vi "Destroy Last Clone Instance Notifier.vi"(11 "Last Instance Notifier":refnum<notifier>) -> ()   [LabVIEW 2019, in "Multiple_uC.lvlib" / "Clone Registration.lvlib"]
doc: "Destroy the notifier.\n_____\nBased on Delacor QMH Project Template 5.0.0.82."
uses:
  Clone Registration.lvlib
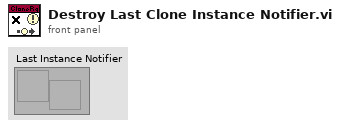
[diagram p1: front panel]
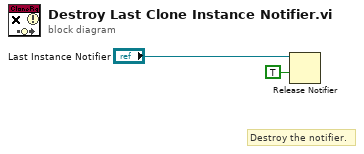
[diagram p0: block diagram]
diagram:
  # "Destroy the notifier."
  n1 = Release Notifier(notifier="Last Instance Notifier", force destroy? (F)=TRUE) -> ()  [unwired: 1 in, 3 out]
